vi "run.vi"(8 "error in (no error)":errorcluster, 10 "control references":T1, 11 "HelioUpdateMH100803 in":refnum<class "HelioUpdateMH100803.lvclass">) -> (0 "error out":errorcluster, 3 "HelioUpdateMH100803 out":refnum<class "HelioUpdateMH100803.lvclass">, 5 "update out":T2)   [LabVIEW 2017, in "HelioUpdateMH100803.lvclass"]
uses:
  HelioUpdateMH100803.lvclass
  main/labview_source/controls/update_picture.ctl
  main/labview_source/type_definitions/clusters/controls_refs.ctl
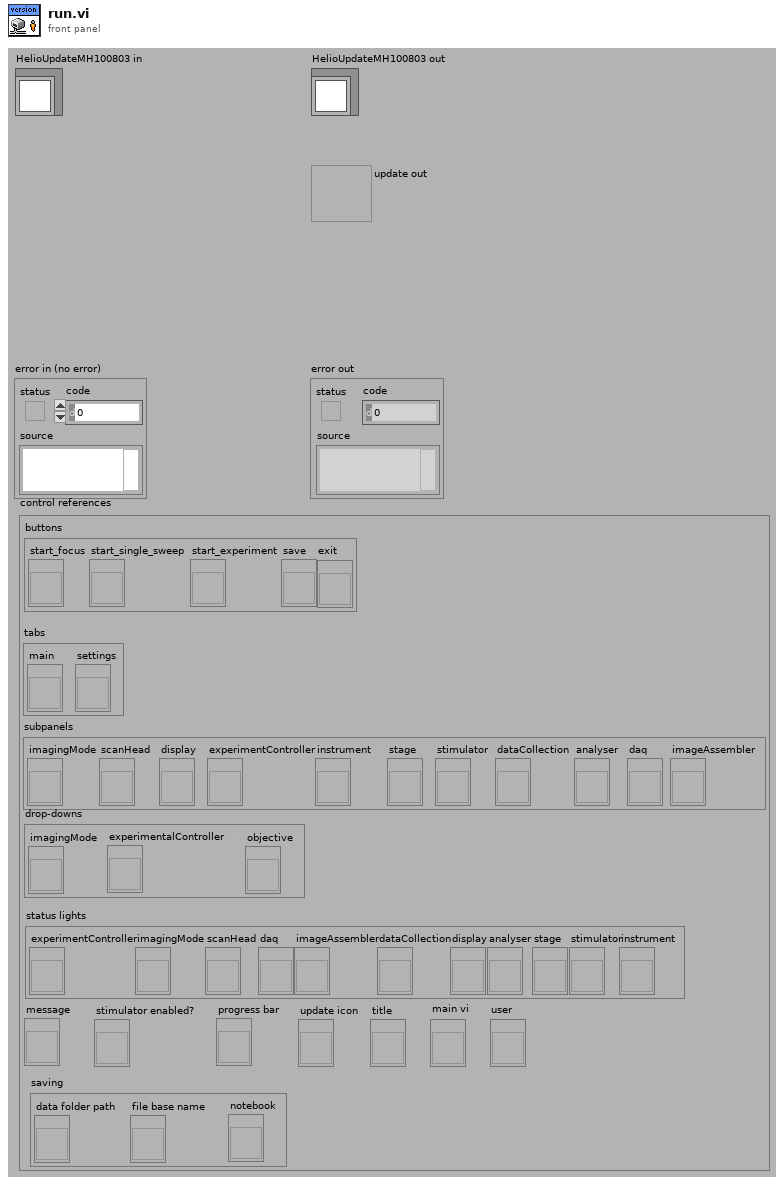
[diagram p1: front panel]
types:
  T1 = typedef "controls_refs.ctl" = cluster{"buttons":cluster{"start_focus":refnum<vi>, "start_single_sweep":refnum<vi>, "start_experiment":refnum<vi>, "save":refnum<vi>, "exit":refnum<vi>}, "tabs":cluster{"main":refnum<vi>, "settings":refnum<vi>}, "subpanels":cluster{"imagingMode":refnum<vi>, "scanHead":refnum<vi>, "display":refnum<vi>, "experimentController":refnum<vi>, "instrument":refnum<vi>, "stage":refnum<vi>, "stimulator":refnum<vi>, "dataCollection":refnum<vi>, "analyser":refnum<vi>, "daq":refnum<vi>, "imageAssembler":refnum<vi>}, "drop-downs":cluster{"imagingMode":refnum<vi>, "experimentalController":refnum<vi>, "objective":refnum<vi>}, "status lights":cluster{"experimentController":refnum<vi>, "imagingMode":refnum<vi>, "scanHead":refnum<vi>, "daq":refnum<vi>, "imageAssembler":refnum<vi>, "dataCollection":refnum<vi>, "display":refnum<vi>, "analyser":refnum<vi>, "stage":refnum<vi>, "stimulator":refnum<vi>, "instrument":refnum<vi>}, "message":refnum<vi>, "stimulator enabled?":refnum<vi>, "saving":cluster{"data folder path":refnum<vi>, "file base name":refnum<vi>, "notebook":refnum<vi>}, "progress bar":refnum<vi>, "update icon":refnum<vi>, "title":refnum<vi>, "main vi":refnum<vi>, "user":refnum<vi>}
  T2 = typedef "HelioUpdateMH100803.lvclass/update_picture.ctl" = u16
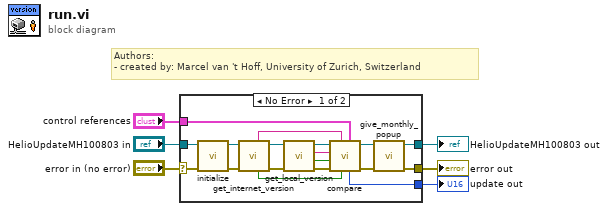
[diagram p0: block diagram]
diagram:
  # "Authors: \n- created by: Marcel van 't Hoff, University of Zurich, Switzerland"
  n1 = case shown="No Error" "error in (no error)" {
    selector: "error in (no error)" -> [w16 w26]
    tunnel: [w8 w26] -> w5
    tunnel: [w7 w25] -> w4
    tunnel: "HelioUpdateMH100803 in" -> [w14 w25]
    tunnel: "control references" -> [w12 _]
    tunnel: [w11 _] -> w1
    frame No Error {
      n2 = call-dynamic "initialize.vi"("error in (no error)"=w16, "HelioUpdateMH100803 in"=w14) -> ("error out"=w15:errorcluster, "HelioUpdateMH100803 out"=w13:refnum<class "HelioUpdateMH100803.lvclass">)  [unwired: 8 in]
      n3 = call-dynamic "get_internet_version.vi"("error in (no error)"=w15, "HelioUpdateMH100803 in"=w13) -> ("error out"=w24:errorcluster, "HelioUpdateMH100803 out"=w23:refnum<class "HelioUpdateMH100803.lvclass">, "version number failed"=w20:bool, "internet version out"=w17:string)  [unwired: 6 in]
      n4 = call-dynamic "get_local_version.vi"("error in (no error)"=w24, "HelioUpdateMH100803 in"=w23) -> ("error out"=w22:errorcluster, "file loading failed?"=w19:bool, "local version out"=w18:string, "HelioUpdateMH100803 out"=w21:refnum<class "HelioUpdateMH100803.lvclass">)  [unwired: 6 in]
      n5 = call-dynamic "compare.vi"("control references"=w12, "internet error?"=w20, "internet version in"=w17, "error in (no error)"=w22, "local error?"=w19, "local version in"=w18, "HelioUpdateMH100803 in"=w21) -> ("error out"=w9:errorcluster, "HelioUpdateMH100803 out"=w10:refnum<class "HelioUpdateMH100803.lvclass">, "update out"=w11:T2)  [unwired: 2 in]
      n6 = call-dynamic "give_monthly_popup.vi"("error in (no error)"=w9, "HelioUpdateMH100803 in"=w10) -> ("error out"=w8:errorcluster, "HelioUpdateMH100803 out"=w7:refnum<class "HelioUpdateMH100803.lvclass">)  [unwired: 8 in]
    }
    frame Error {
    }
  }
  "error out" <- w5
  "HelioUpdateMH100803 out" <- w4
  "update out" <- w1
